vi "sv_Uniquify String.vi"(9 "separator":string="_", 10 "reserved strings":string[](array[string]), 11 "string":string) -> (1 "uniquifier":string, 2 "unique increment":u64, 3 "unique string":string)   [LabVIEW 2017]
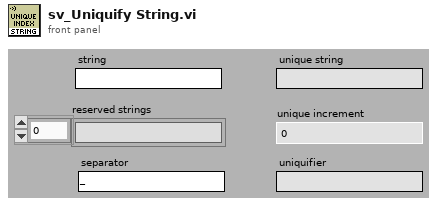
[diagram p1: front panel]
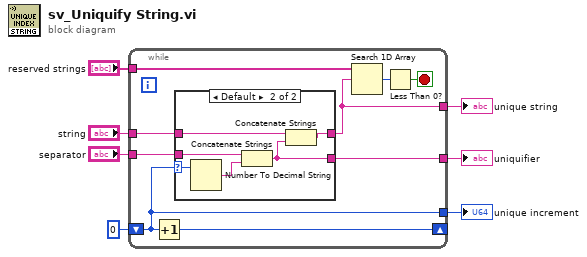
[diagram p0: block diagram]
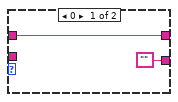
[diagram p2: hidden frame]
diagram:
  n1 = while {
    tunnel: "reserved strings" -> [w16]
    tunnel: [w11] -> w6
    tunnel: "string" -> [w13]
    shift-right: [w12] -> _
    shift-left: u64 0 -> [w9]
    tunnel: "separator" -> [w10]
    tunnel: [w9] -> w2
    tunnel: [w8] -> w1
    stop <- w14 stop-if-true
    n2 = Increment(x=w9) -> (x+1=w12:u64)
    n3 = case shown="Default" w9 {
      selector: w9 -> [_ w23]
      tunnel: w13 -> [w18 w24]
      tunnel: [w18 w21] -> w11
      tunnel: w10 -> [_ w22]
      tunnel: ["" w19] -> w8
      frame 0 {
      }
      frame Default {
        n4 = Number To Decimal String(number=w23) -> (decimal integer string=w20:string)  [unwired: 1 in]
        n5 = Concatenate Strings(w22, w20) -> (w19:string)
        n6 = Concatenate Strings(w24, w19) -> (w21:string)
      }
    }
    n7 = Search 1D Array(1D array=w16, element=w11) -> (index of element=w15:i32)  [unwired: 1 in]
    n8 = Less Than 0?(x=w15) -> (x < 0?=w14:bool)
  }
  "unique string" <- w6
  "uniquifier" <- w1
  "unique increment" <- w2
